vi "ECS-100X-PFI-RT.vi"() -> ()   [LabVIEW 2015]
uses:
  Typedefs/FPGA Refs/Generic FPGA Ref.ctl
  Typedefs/RT Data.ctl
  Typedefs/FPGA Refs/FPGA Refs.ctl
  Typedefs/EPT/EPT Cluster.ctl
  <vilib>/Powertrain Controls/Device Drivers/Engine Position Tracking/EPTx/RevA/RT/Controls/EPTxData.ctl
  Typedefs/Raw Inputs/Raw Inputs.ctl
  Typedefs/Raw Inputs/NI9752.ctl
  Typedefs/Raw Inputs/PPWData.ctl
  Typedefs/Raw Inputs/NI9757.ctl
  Typedefs/Raw Inputs/NI9411.ctl
  Typedefs/Raw Inputs/NI9220.ctl
  Typedefs/Raw Inputs/VRHall.ctl
  Typedefs/Control Inputs/Control Inputs.ctl
  Typedefs/EPT/Engine Status.ctl
  Typedefs/MISC/Load Control Mode.ctl
  Typedefs/Control Outputs/Control Outputs.ctl
  Typedefs/Control Outputs/Injection Quantity.ctl
  Typedefs/Control Outputs/Injection Timing.ctl
  Typedefs/Raw Outputs/Raw Outputs.ctl
  Typedefs/Raw Outputs/NI9751.ctl
  Typedefs/Raw Outputs/DI.ctl
  Typedefs/Raw Outputs/NI9754.ctl
  Typedefs/Raw Outputs/ESTTL.ctl
  Typedefs/Raw Outputs/NI9758.ctl
  Typedefs/Raw Outputs/LS.ctl
  Typedefs/Raw Outputs/PFI.ctl
  Typedefs/Raw Outputs/NI9759.ctl
  <vilib>/Platform/TimedLoop/XDataNode/timing_clust.ctl
  <vilib>/Platform/TimedLoop/XDataNode/nitl_modes.ctl
  <vilib>/Platform/TimedLoop/XDataNode/wakeup.ctl
  <vilib>/addons/Combustion Analysis System/Real-Time/Controls/Settings/CAS - Settings - Slow Speed Data.ctl
  <vilib>/addons/Combustion Analysis System/FPGA/CAS - FGPA - Reference.ctl
  Globals/DIScope Globals.vi
  <vilib>/FPGAPlugInAG/PXI-7853R/niLvFpga_Open_PXI-7853R.vi
  <vilib>/rvi/interface/common/dynamic/niFpgaDynamicAddResources.vi
  <vilib>/addons/Combustion Analysis System/Real-Time/Globals/CAS - Slow Speed Data.vi
  <vilib>/addons/Combustion Analysis System/Real-Time/Globals/Settings/CAS - Settings - Custom Properties.vi
  Globals/RT Data.vi
  <vilib>/rvi/interface/nirviOpenFPGA/nirviOpenFPGA.xnode
  FPGA Bitfiles/ECS-100X-FPGA1-EPTx.lvbitx
  FPGA Bitfiles/ECS-100X-FPGA2-EPTx.lvbitx
  <vilib>/Platform/TimedLoop/XDataNode/XDataNode.xnode
  ECS-RT.lvlib
  <vilib>/Platform/TimedLoop/XDataNode/XDNodeRunTimeDep.lvlib
  ECS-Shared.lvlib
  <vilib>/Powertrain Controls/Device Drivers/Engine Position Tracking/EPTx/RevA/RT/EPTx - RevA - RT.lvlib
panel:
  out "System Loop Iteration":i32
  in  "Stop RT":bool
  out "FPGA 2":errorcluster
  out "Slow Speed Loop Iteration":i32
  out "Iteration Duration":i64
  out "SCMInitOK":bool
  out "FPGA 1":errorcluster
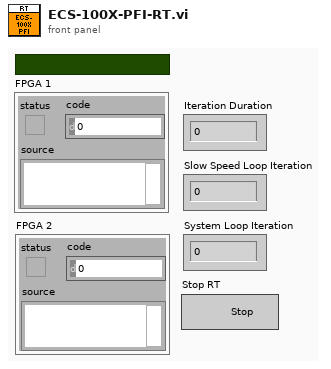
[diagram p1: front panel]
types:
  T1 = typedef "ECS-Shared.lvlib/RT Data.ctl" = cluster{"Refs":T2, "EPT":T4, "Raw Inputs":T6, "Control Inputs":T13, "Control Outputs":T16, "Raw Outputs":T19}
  T2 = typedef "ECS-Shared.lvlib/FPGA Refs.ctl" = cluster{"FPGA 1":T3, "FPGA 2":T3}
  T3 = typedef "ECS-Shared.lvlib/Generic FPGA Ref.ctl" = refnum<k20>
  T4 = typedef "ECS-Shared.lvlib/EPT Cluster.ctl" = cluster{"MaxCAD":sgl, "EPT Sim Enabled":bool, "EPTxData":T5}
  T5 = typedef "EPTx - RevA - RT.lvlib/EPTxData.ctl" = cluster{"Sync":bool, "CurrentCAD":sgl, "Speed [RPM]":sgl, "Config":bool, "Rcvg Primary":bool, "Stall":bool, "Overflow":bool, "Ratio Error":bool, "Pattern Error":bool, "Aux Warning":bool, "Watchdog Error":bool}
  T6 = typedef "ECS-Shared.lvlib/Raw Inputs.ctl" = cluster{"NI9752s":T7[], "NI9757s":T9[], "NI9411s":T10[], "NI9220s":T11[], "VRHalls":T12[]}
  T7 = typedef "ECS-Shared.lvlib/NI9752.ctl" = cluster{"Voltage [V]":sgl[], "Resistance [Ohm]":sgl[], "PPWData VR1":T8, "PPWData VR2":T8, "PPWData Hall1":T8, "PPWData Hall2":T8}
  T8 = typedef "ECS-Shared.lvlib/PPWData.ctl" = cluster{"Period":u32, "PulseWidth":u32, "Stopped":bool}
  T9 = typedef "ECS-Shared.lvlib/NI9757.ctl" = cluster{"UEGO1":cluster{"Lambda":sgl, "Phi":sgl, "AF_Ratio":sgl, "Ip":sgl, "Temp":sgl, "Hot":bool}, "UEGO2":cluster{"Lambda":sgl, "Phi":sgl, "AF_Ratio":sgl, "Ip":sgl, "Temp":sgl, "Hot":bool}, "EGO1":cluster{"Status":enum16{"COLD SENSOR", "FOULED SENSOR", "RICH", "LEAN"}, "SensorV":sgl}, "EGO2":cluster{"Status":enum16{"COLD SENSOR", "FOULED SENSOR", "RICH", "LEAN"}, "SensorV":sgl}, "EGO3":cluster{"Status":enum16{"COLD SENSOR", "FOULED SENSOR", "RICH", "LEAN"}, "SensorV":sgl}, "EGO4":cluster{"Status":enum16{"COLD SENSOR", "FOULED SENSOR", "RICH", "LEAN"}, "SensorV":sgl}}
  T10 = typedef "ECS-Shared.lvlib/NI9411.ctl" = cluster{"PPWData 0":T8, "PPWData 1":T8, "PPWData 2":T8, "PPWData 3":T8, "PPWData 4":T8, "PPWData 5":T8}
  T11 = typedef "ECS-Shared.lvlib/NI9220.ctl" = cluster{"AI 0":sgl, "AI 1":sgl, "AI 2":sgl, "AI 3":sgl, "AI 4":sgl, "AI 5":sgl, "AI 6":sgl, "AI 7":sgl, "AI 8":sgl, "AI 9":sgl, "AI 10":sgl, "AI 11":sgl, "AI 12":sgl, "AI 13":sgl, "AI 14":sgl, "AI 15":sgl}
  T12 = typedef "ECS-Shared.lvlib/VRHall.ctl" = cluster{"PPWData 0":T8, "PPWData 1":T8, "PPWData 2":T8, "PPWData 3":T8, "PPWData 4":T8, "PPWData 5":T8}
  T13 = typedef "ECS-Shared.lvlib/Control Inputs.ctl" = cluster{"Engine Speed [RPM]":sgl, "Engine Status":T14, "Load Control \nMode":T15, "dt(s)":sgl, "Number of Cylinders":u8, "Engine Displacement [cc]":sgl, "StoichAFR":sgl, "Q.LHV Fuel [kJ/kg]":sgl, "BattV PSU [V]":sgl, "12V PSU [V]":sgl, "5V PSU [V]":sgl, "Pedal Position [%]":sgl, "Oil Pressure [kPa]":sgl, "Oil Temp [C]":sgl, "Oil Level [%]":sgl, "Engine Coolant Temp (ECT) [C]":sgl, "Engine Coolant Pressure [kPa]":sgl, "Rail Pressure [bar]":sgl, "Fuel Pressure [kPa]":sgl, "Fuel Temp [C]":sgl, "Vacuum Pressure [kPa]":sgl, "Throttle Position [%]":sgl, "Cam1 Advance [CAD]":sgl, "Cam2 Advance [CAD]":sgl, "Cam3 Advance [CAD]":sgl, "Cam4 Advance [CAD]":sgl, "CA50 Control Output [CAD]":sgl[], "CA50 Control Output Valid":bool[], "Intake Air Temp (IAT) [C]":sgl, "Barometric Air Pressure [kPa]":sgl, "Intake Air Rel. Humidity [%]":sgl, "Mass Air Flow (MAF) [kg/hr]":sgl, "Turbo Inlet Air Pressure [kPa]":sgl, "Turbo Inlet Air Temp [C]":sgl, "Turbo Outlet Air Pressure [kPa]":sgl, "Turbo Outlet Air Temp [C]":sgl, "CAC Outlet Pressure [kPa]":sgl, "CAC Outlet Temp [C]":sgl, "Intake Manifold Pressure (MAP) [kPa]":sgl, "Intake Manifold Temp (MAT) [C]":sgl, "Exhaust Manifold Pressure [kPa]":sgl, "Exhaust Manifold Temp [C]":sgl, "HighP EGR Cooler Outlet Pressure [kPa]":sgl, "HighP EGR Cooler Outlet Temp [C]":sgl, "HighP EGR Differential Pressure [kPa]":sgl, "HighP EGR Valve Position [%]":sgl, "Turbo Outlet Exhaust Pressure [kPa]":sgl, "Turbo Outlet Exhaust Temp [C]":sgl, "VGT Position 1 [%]":sgl, "VGT Position 2 [%]":sgl, "Turbo Speed 1 [RPM]":sgl, "Turbo Speed 2 [RPM]":sgl, "LowP EGR Differential Pressure [kPa]":sgl, "LowP EGR Valve Position [%]":sgl, "UEGO1Lambda":sgl, "UEGO1_Hot":bool, "UEGO2Lambda":sgl, "UEGO2_Hot":bool, "Knock Intensity":sgl[], "Knock":bool[]}
  T14 = typedef "ECS-Shared.lvlib/Engine Status.ctl" = enum16{"OFF", "STALLED", "CRANKING", "RUNNING", "ACCEL", "DECEL", "SAFE"}
  T15 = typedef "ECS-Shared.lvlib/Load Control Mode.ctl" = enum16{"No Governor", "Low-Idle Governor", "High-Idle Governor"}
  T16 = typedef "ECS-Shared.lvlib/Control Outputs.ctl" = cluster{"Pedal Desired [%]":sgl, "MEP Desired [bar]":sgl, "Fuel Desired [mg/cyc]":sgl, "Intake MAP Desired [kPa]":sgl, "Cam1 Advance Setpoint [CAD]":sgl, "Cam2 Advance Setpoint [CAD]":sgl, "HighP EGR Position Setpoint [%Open]":sgl, "LowP EGR Position Setpoint [%Open]":sgl, "Rail Pressure Setpoint [bar]":sgl, "Wastegate1 Position Setpoint [%Open]":sgl, "Wastegate2 Position Setpoint [%Open]":sgl, "VGT1 Position Setpoint [%Open]":sgl, "VGT2 Position Setpoint [%Open]":sgl, "Throttle1 Position Setpoint [%Open]":sgl, "Throttle2 Position Setpoint [%Open]":sgl, "TurboBPV Position Setpoint [%Open]":sgl, "Spark Dwells [msec]":sgl[], "Spark Timings [DBTDC]":sgl[], "PFI Quantities [mg/inj]":sgl[], "PFI Timings [DBTDC]":sgl[], "DI Quantities [mg/inj]":T17[], "DI Timings [DBTDC]":T18[]}
  T17 = typedef "ECS-Shared.lvlib/Injection Quantity.ctl" = cluster{"Pilot1Quantity [mg/inj]":sgl, "Pilot2Quantity [mg/inj]":sgl, "MainQuantity [mg/inj]":sgl, "Post1Quantity [mg/inj]":sgl, "Post2Quantity [mg/inj]":sgl}
  T18 = typedef "ECS-Shared.lvlib/Injection Timing.ctl" = cluster{"Pilot1SOI [DBTDC]":sgl, "Pilot2SOI [DBTDC]":sgl, "MainSOI [DBTDC]":sgl, "Post1SOI [DBTDC]":sgl, "Post2SOI [DBTDC]":sgl}
  T19 = typedef "ECS-Shared.lvlib/Raw Outputs.ctl" = cluster{"9751-1":T20, "9751-2":T20, "9751-3":T20, "9751-4":T20, "9754-1":T22, "9754-2":T22, "9758-1":T24, "9758-2":T24, "9759-1":T27}
  T20 = typedef "ECS-Shared.lvlib/NI9751.ctl" = cluster{"DI1":T21, "DI2":T21, "DI3":T21}
  T21 = typedef "ECS-Shared.lvlib/DI.ctl" = cluster{"Window_Start (DBTDC)":sgl, "Window_End (DBTDC)":sgl, "Enable_Inj1":bool, "Duration_Inj1 (msec)":sgl, "Timing_Inj1 (DBTDC)":sgl, "Enable_Inj2":bool, "Duration_Inj2 (msec)":sgl, "Timing_Inj2 (DBTDC)":sgl, "Enable_Inj3":bool, "Duration_Inj3 (msec)":sgl, "Timing_Inj3 (DBTDC)":sgl, "Enable_Inj4":bool, "Duration_Inj4 (msec)":sgl, "Timing_Inj4 (DBTDC)":sgl, "Enable_Inj5":bool, "Duration_Inj5 (msec)":sgl, "Timing_Inj5 (DBTDC)":sgl}
  T22 = typedef "ECS-Shared.lvlib/NI9754.ctl" = cluster{"ESTTL 1":T23, "ESTTL 2":T23, "ESTTL 3":T23, "ESTTL 4":T23, "ESTTL 5":T23, "ESTTL 6":T23, "ESTTL 7":T23, "ESTTL 8":T23}
  T23 = typedef "ECS-Shared.lvlib/ESTTL.ctl" = cluster{"Timing (DBTDC)":sgl, "Dwell (ms)":sgl}
  T24 = typedef "ECS-Shared.lvlib/NI9758.ctl" = cluster{"LS 1":T25, "LS 2":T25, "LS 3":T25, "LS 4":T25, "PFI 1":T26, "PFI 2":T26, "PFI 3":T26, "PFI 4":T26}
  T25 = typedef "ECS-Shared.lvlib/LS.ctl" = cluster{"Enable":bool, "Freq [Hz]":sgl, "DutyCyc [%]":sgl}
  T26 = typedef "ECS-Shared.lvlib/PFI.ctl" = cluster{"Position Mode":bool, "Timing (DBTDC)":sgl, "Pulse Width (ms)":sgl}
  T27 = typedef "ECS-Shared.lvlib/NI9759.ctl" = cluster{"THR1-1 DC [%]":sgl, "THR1-1 Setpoint [% Open]":sgl, "THR1-2 DC [%]":sgl, "THR1-2 Setpoint [% Open]":sgl}
  T28 = typedef "CAS - FGPA - Reference.ctl" = refnum<k20>
  T29 = typedef "XDNodeRunTimeDep.lvlib/timing_clust.ctl" = cluster{"Expected End [f-1]":u64, "Actual End [f-1]":u64, "Finished Late? [f-1]":bool, "Expected End [i-1]":u64, "Actual End [i-1]":u64, "Finished Late? [i-1]":bool, "Expected Start [i]":u64, "Actual Start [i]":u64, "Expected Start [f]":u64, "Actual Start [f]":u64, "Source Name":string, "Structure Name":string, "Period":i64, "Deadline":i64, "Offset":i64, "Start":i64, "Priority":i32, "Timeout":i32, "Mode":T30, "Wakeup Reason":T31, "Error":errorcluster, "Source Type":string, "Secondary Source Type":string, "Global End Time":u64, "Global Start Time":u64, "Frame Duration":u64, "Iteration Duration":u64, "Assigned CPU":i32, "I/O Scan Engine Mode":u32}
  T30 = typedef "XDNodeRunTimeDep.lvlib/nitl_modes.ctl" = enum32{"No Change", "Process missed periods, maintain original phase", "Discard missed periods, maintain original phase", "Process missed periods, ignore original phase", "Discard missed periods, ignore original phase"}
  T31 = typedef "XDNodeRunTimeDep.lvlib/wakeup.ctl" = enum32{"Normal", "Aborted", "Asynchronous wakeup", "Timing source error", "Timed loop error", "Timeout"}
  T32 = typedef "CAS - Settings - Slow Speed Data.ctl" = cluster{"Name":string, "Units":string, "Value":sgl}
  T33 = typedef "CAS - Settings - Custom Properities.ctl" = T34[]
  T34 = typedef "CAS - Settings - Custom Properity.ctl" = cluster{"Properity":string, "Data":string}
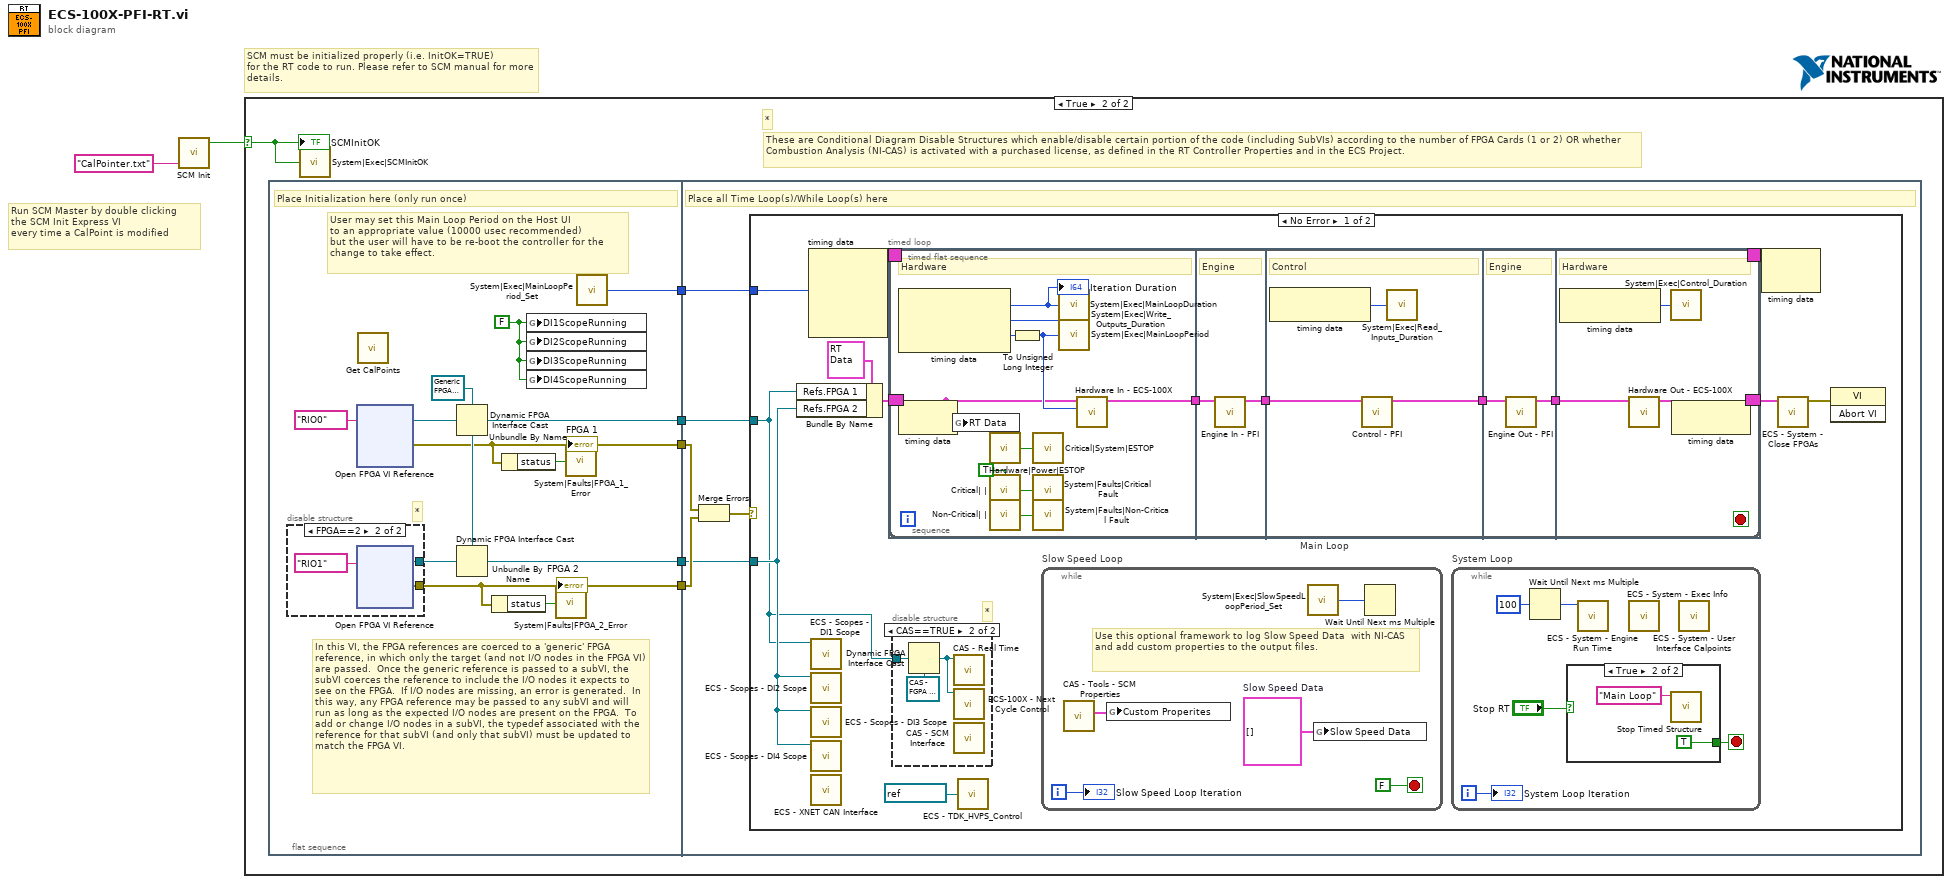
[diagram p0: block diagram]
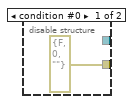
[diagram p3: hidden frame]
diagram:
  # "SCM must be initialized properly (i.e. InitOK=TRUE)\nfor the RT code to run. Please refer to SCM manual for more details."
  # "Run SCM Master by double clicking\nthe SCM Init Express VI\nevery time a CalPoint is modified"
  n1 = call "SCM Init"("Calibration File"="CalPointer.txt") -> ("InitOK"=w2:bool)  [unwired: 2 in, 2 out]
  n2 = case shown="True" w2 {
    selector: w2 -> [_ w8]
    frame False {
    }
    frame True {
      # "These are Conditional Diagram Disable Structures which enable/disable certain portion of the code (including SubVIs) according to the number of FPGA Cards (1 or 2) OR whether Combustion Analysis (NI-CAS) is activated with a purchased license, as defined in the RT Controller Properties and in the ECS Project."
      # "*"
      n3 = flat-sequence {
        tunnel: [w9] -> w7
        tunnel: [w16] -> w6
        tunnel: [w19] -> w5
        tunnel: [w15] -> w4
        tunnel: [w12] -> w3
        tunnel: w7 -> [w30]
        tunnel: w6 -> [w29]
        tunnel: w5 -> [w27]
        tunnel: w4 -> [w26]
        tunnel: w3 -> [w25]
        frame #0 {
          w13 = T3 refnum ("FPGA VI Reference Out")
          w18 = FALSE ("DIScopeTransfer")
          # "*"
          # "In this VI, the FPGA references are coerced to a 'generic' FPGA reference, in which only the target (and not I/O nodes in the FPGA VI) are passed.  Once the generic reference is passed to a subVI, the subVI coerces the reference to include the I/O nodes it expects to see on the FPGA.  If I/O nodes are missing, an error is generated.  In this way, any FPGA reference may be passed to any subVI and will run as long as the expected I/O nodes are present on the FPGA.  To add or change I/O nodes in a subVI, the typedef associated with the reference for that subVI (and only that subVI) must be updated to match the FPGA VI."
          # "User may set this Main Loop Period on the Host UI\nto an appropriate value (10000 usec recommended)\nbut the user will have to be re-boot the controller for the\nchange to take effect."
          # "Place Initialization here (only run once)"
          n4 = disable-structure shown="FPGA==2" {
            disable-tunnel: [errorcluster {"status"=FALSE, "code"=0, "source"=""} ("error out") w23] -> w16
            disable-tunnel: [_ w22] -> w14
            frame condition #0 {
            }
            frame condition #1 (active) {
              n5 = xnode "Open FPGA VI Reference"("resource name"=tag "RIO1") -> ("FPGA VI Reference Out"=w22:refnum<k20>, "error out"=w23:errorcluster)  [unwired: 1 in]
            }
          }
          "FPGA 2" <- w16
          n6 = xnode "Open FPGA VI Reference"("resource name"=tag "RIO0") -> ("FPGA VI Reference Out"=w10:refnum<k20>, "error out"=w9:errorcluster)  [unwired: 1 in]
          "FPGA 1" <- w9
          n7 = call "Get CalPoints.vi"() -> ()  [unwired: 12 in]
          n8 = Dynamic FPGA Interface Cast(Session In=w13, Type=w10) -> (Session Out=w15:T3)
          n9 = Dynamic FPGA Interface Cast(Session In=w13, Type=w14) -> (Session Out=w12:T3)
          n10 = Unbundle By Name(w16) -> ("status"=w17:bool)
          n11 = Unbundle By Name(w9) -> ("status"=w20:bool)
          n12 = global write "DIScope Globals.vi" "DI1ScopeRunning"(w18) -> ()
          n13 = global write "DIScope Globals.vi" "DI2ScopeRunning"(w18) -> ()
          n14 = global write "DIScope Globals.vi" "DI3ScopeRunning"(w18) -> ()
          n15 = global write "DIScope Globals.vi" "DI4ScopeRunning"(w18) -> ()
          n16 = call "System|Faults|FPGA_2_Error"("Value"=w17) -> ()
          n17 = call "System|Faults|FPGA_1_Error"("Value"=w20) -> ()
          n18 = call "System|Exec|MainLoopPeriod_Set"() -> ("Value"=w19:u32)
        }
        frame #1 {
          # "Place all Time Loop(s)/While Loop(s) here"
          n19 = Merge Errors(w30, w29) -> (w28:errorcluster)
          n20 = case shown="No Error" w28 {
            tunnel: w27 -> [w38 _]
            tunnel: w26 -> [w33 _]
            tunnel: w25 -> [w35 _]
            frame No Error {
              # "*"
              n21 = Bundle By Name(cluster=T1 {"Refs"={"FPGA 1"=refnum, "FPGA 2"=refnum}, "EPT"={"MaxCAD"=0.0, "EPT Sim Enabled"=FALSE, "EPTxData"={"Sync"=FALSE, "CurrentCAD"=0.0, "Speed [RPM]"=0.0, "Config"=FALSE, "Rcvg Primary"=FALSE, "Stall"=FALSE, "Overflow"=FALSE, "Ratio Error"=FALSE, "Pattern Error"=FALSE, "Aux Warning"=FALSE, "Watchdog Error"=FALSE}}, "Raw Inputs"={"NI9752s"=[], "NI9757s"=[], "NI9411s"=[], "NI9220s"=[], "VRHalls"=[]}, "Control Inputs"={"Engine Speed [RPM]"=0.0, "Engine Status"=enum."STALLED", "Load Control \nMode"=enum."No Governor", "dt(s)"=0.0, "Number of Cylinders"=0, "Engine Displacement [cc]"=0.0, "StoichAFR"=0.0, "Q.LHV Fuel [kJ/kg]"=0.0, "BattV PSU [V]"=0.0, "12V PSU [V]"=0.0, "5V PSU [V]"=0.0, "Pedal Position [%]"=0.0, "Oil Pressure [kPa]"=0.0, "Oil Temp [C]"=0.0, "Oil Level [%]"=0.0, "Engine Coolant Temp (ECT) [C]"=0.0, "Engine Coolant Pressure [kPa]"=0.0, "Rail Pressure [bar]"=0.0, "Fuel Pressure [kPa]"=0.0, "Fuel Temp [C]"=0.0, "Vacuum Pressure [kPa]"=0.0, "Throttle Position [%]"=0.0, "Cam1 Advance [CAD]"=0.0, "Cam2 Advance [CAD]"=0.0, "Cam3 Advance [CAD]"=0.0, "Cam4 Advance [CAD]"=0.0, "CA50 Control Output [CAD]"=[], "CA50 Control Output Valid"=[], "Intake Air Temp (IAT) [C]"=0.0, "Barometric Air Pressure [kPa]"=0.0, "Intake Air Rel. Humidity [%]"=0.0, "Mass Air Flow (MAF) [kg/hr]"=0.0, "Turbo Inlet Air Pressure [kPa]"=0.0, "Turbo Inlet Air Temp [C]"=0.0, "Turbo Outlet Air Pressure [kPa]"=0.0, "Turbo Outlet Air Temp [C]"=0.0, "CAC Outlet Pressure [kPa]"=0.0, "CAC Outlet Temp [C]"=0.0, "Intake Manifold Pressure (MAP) [kPa]"=0.0, "Intake Manifold Temp (MAT) [C]"=0.0, "Exhaust Manifold Pressure [kPa]"=0.0, "Exhaust Manifold Temp [C]"=0.0, "HighP EGR Cooler Outlet Pressure [kPa]"=0.0, "HighP EGR Cooler Outlet Temp [C]"=0.0, "HighP EGR Differential Pressure [kPa]"=0.0, "HighP EGR Valve Position [%]"=0.0, "Turbo Outlet Exhaust Pressure [kPa]"=0.0, "Turbo Outlet Exhaust Temp [C]"=0.0, "VGT Position 1 [%]"=0.0, "VGT Position 2 [%]"=0.0, "Turbo Speed 1 [RPM]"=0.0, "Turbo Speed 2 [RPM]"=0.0, "LowP EGR Differential Pressure [kPa]"=0.0, "LowP EGR Valve Position [%]"=0.0, "UEGO1Lambda"=0.0, "UEGO1_Hot"=FALSE, "UEGO2Lambda"=0.0, "UEGO2_Hot"=FALSE, "Knock Intensity"=[], "Knock"=[]}, "Control Outputs"={"Pedal Desired [%]"=0.0, "MEP Desired [bar]"=0.0, "Fuel Desired [mg/cyc]"=0.0, "Intake MAP Desired [kPa]"=0.0, "Cam1 Advance Setpoint [CAD]"=0.0, "Cam2 Advance Setpoint [CAD]"=0.0, "HighP EGR Position Setpoint [%Open]"=0.0, "LowP EGR Position Setpoint [%Open]"=0.0, "Rail Pressure Setpoint [bar]"=0.0, "Wastegate1 Position Setpoint [%Open]"=0.0, "Wastegate2 Position Setpoint [%Open]"=0.0, "VGT1 Position Setpoint [%Open]"=0.0, "VGT2 Position Setpoint [%Open]"=0.0, "Throttle1 Position Setpoint [%Open]"=0.0, "Throttle2 Position Setpoint [%Open]"=0.0, "TurboBPV Position Setpoint [%Open]"=0.0, "Spark Dwells [msec]"=[], "Spark Timings [DBTDC]"=[], "PFI Quantities [mg/inj]"=[], "PFI Timings [DBTDC]"=[], "DI Quantities [mg/inj]"=[], "DI Timings [DBTDC]"=[]}, "Raw Outputs"={"9751-1"={"DI1"={"Window_Start (DBTDC)"=0.0, "Window_End (DBTDC)"=0.0, "Enable_Inj1"=FALSE, "Duration_Inj1 (msec)"=0.0, "Timing_Inj1 (DBTDC)"=0.0, "Enable_Inj2"=FALSE, "Duration_Inj2 (msec)"=0.0, "Timing_Inj2 (DBTDC)"=0.0, "Enable_Inj3"=FALSE, "Duration_Inj3 (msec)"=0.0, "Timing_Inj3 (DBTDC)"=0.0, "Enable_Inj4"=FALSE, "Duration_Inj4 (msec)"=0.0, "Timing_Inj4 (DBTDC)"=0.0, "Enable_Inj5"=FALSE, "Duration_Inj5 (msec)"=0.0, "Timing_Inj5 (DBTDC)"=0.0}, "DI2"={"Window_Start (DBTDC)"=0.0, "Window_End (DBTDC)"=0.0, "Enable_Inj1"=FALSE, "Duration_Inj1 (msec)"=0.0, "Timing_Inj1 (DBTDC)"=0.0, "Enable_Inj2"=FALSE, "Duration_Inj2 (msec)"=0.0, "Timing_Inj2 (DBTDC)"=0.0, "Enable_Inj3"=FALSE, "Duration_Inj3 (msec)"=0.0, "Timing_Inj3 (DBTDC)"=0.0, "Enable_Inj4"=FALSE, "Duration_Inj4 (msec)"=0.0, "Timing_Inj4 (DBTDC)"=0.0, "Enable_Inj5"=FALSE, "Duration_Inj5 (msec)"=0.0, "Timing_Inj5 (DBTDC)"=0.0}, "DI3"={"Window_Start (DBTDC)"=0.0, "Window_End (DBTDC)"=0.0, "Enable_Inj1"=FALSE, "Duration_Inj1 (msec)"=0.0, "Timing_Inj1 (DBTDC)"=0.0, "Enable_Inj2"=FALSE, "Duration_Inj2 (msec)"=0.0, "Timing_Inj2 (DBTDC)"=0.0, "Enable_Inj3"=FALSE, "Duration_Inj3 (msec)"=0.0, "Timing_Inj3 (DBTDC)"=0.0, "Enable_Inj4"=FALSE, "Duration_Inj4 (msec)"=0.0, "Timing_Inj4 (DBTDC)"=0.0, "Enable_Inj5"=FALSE, "Duration_Inj5 (msec)"=0.0, "Timing_Inj5 (DBTDC)"=0.0}}, "9751-2"={"DI1"={"Window_Start (DBTDC)"=0.0, "Window_End (DBTDC)"=0.0, "Enable_Inj1"=FALSE, "Duration_Inj1 (msec)"=0.0, "Timing_Inj1 (DBTDC)"=0.0, "Enable_Inj2"=FALSE, "Duration_Inj2 (msec)"=0.0, "Timing_Inj2 (DBTDC)"=0.0, "Enable_Inj3"=FALSE, "Duration_Inj3 (msec)"=0.0, "Timing_Inj3 (DBTDC)"=0.0, "Enable_Inj4"=FALSE, "Duration_Inj4 (msec)"=0.0, "Timing_Inj4 (DBTDC)"=0.0, "Enable_Inj5"=FALSE, "Duration_Inj5 (msec)"=0.0, "Timing_Inj5 (DBTDC)"=0.0}, "DI2"={"Window_Start (DBTDC)"=0.0, "Window_End (DBTDC)"=0.0, "Enable_Inj1"=FALSE, "Duration_Inj1 (msec)"=0.0, "Timing_Inj1 (DBTDC)"=0.0, "Enable_Inj2"=FALSE, "Duration_Inj2 (msec)"=0.0, "Timing_Inj2 (DBTDC)"=0.0, "Enable_Inj3"=FALSE, "Duration_Inj3 (msec)"=0.0, "Timing_Inj3 (DBTDC)"=0.0, "Enable_Inj4"=FALSE, "Duration_Inj4 (msec)"=0.0, "Timing_Inj4 (DBTDC)"=0.0, "Enable_Inj5"=FALSE, "Duration_Inj5 (msec)"=0.0, "Timing_Inj5 (DBTDC)"=0.0}, "DI3"={"Window_Start (DBTDC)"=0.0, "Window_End (DBTDC)"=0.0, "Enable_Inj1"=FALSE, "Duration_Inj1 (msec)"=0.0, "Timing_Inj1 (DBTDC)"=0.0, "Enable_Inj2"=FALSE, "Duration_Inj2 (msec)"=0.0, "Timing_Inj2 (DBTDC)"=0.0, "Enable_Inj3"=FALSE, "Duration_Inj3 (msec)"=0.0, "Timing_Inj3 (DBTDC)"=0.0, "Enable_Inj4"=FALSE, "Duration_Inj4 (msec)"=0.0, "Timing_Inj4 (DBTDC)"=0.0, "Enable_Inj5"=FALSE, "Duration_Inj5 (msec)"=0.0, "Timing_Inj5 (DBTDC)"=0.0}}, "9751-3"={"DI1"={"Window_Start (DBTDC)"=0.0, "Window_End (DBTDC)"=0.0, "Enable_Inj1"=FALSE, "Duration_Inj1 (msec)"=0.0, "Timing_Inj1 (DBTDC)"=0.0, "Enable_Inj2"=FALSE, "Duration_Inj2 (msec)"=0.0, "Timing_Inj2 (DBTDC)"=0.0, "Enable_Inj3"=FALSE, "Duration_Inj3 (msec)"=0.0, "Timing_Inj3 (DBTDC)"=0.0, "Enable_Inj4"=FALSE, "Duration_Inj4 (msec)"=0.0, "Timing_Inj4 (DBTDC)"=0.0, "Enable_Inj5"=FALSE, "Duration_Inj5 (msec)"=0.0, "Timing_Inj5 (DBTDC)"=0.0}, "DI2"={"Window_Start (DBTDC)"=0.0, "Window_End (DBTDC)"=0.0, "Enable_Inj1"=FALSE, "Duration_Inj1 (msec)"=0.0, "Timing_Inj1 (DBTDC)"=0.0, "Enable_Inj2"=FALSE, "Duration_Inj2 (msec)"=0.0, "Timing_Inj2 (DBTDC)"=0.0, "Enable_Inj3"=FALSE, "Duration_Inj3 (msec)"=0.0, "Timing_Inj3 (DBTDC)"=0.0, "Enable_Inj4"=FALSE, "Duration_Inj4 (msec)"=0.0, "Timing_Inj4 (DBTDC)"=0.0, "Enable_Inj5"=FALSE, "Duration_Inj5 (msec)"=0.0, "Timing_Inj5 (DBTDC)"=0.0}, "DI3"={"Window_Start (DBTDC)"=0.0, "Window_End (DBTDC)"=0.0, "Enable_Inj1"=FALSE, "Duration_Inj1 (msec)"=0.0, "Timing_Inj1 (DBTDC)"=0.0, "Enable_Inj2"=FALSE, "Duration_Inj2 (msec)"=0.0, "Timing_Inj2 (DBTDC)"=0.0, "Enable_Inj3"=FALSE, "Duration_Inj3 (msec)"=0.0, "Timing_Inj3 (DBTDC)"=0.0, "Enable_Inj4"=FALSE, "Duration_Inj4 (msec)"=0.0, "Timing_Inj4 (DBTDC)"=0.0, "Enable_Inj5"=FALSE, "Duration_Inj5 (msec)"=0.0, "Timing_Inj5 (DBTDC)"=0.0}}, "9751-4"={"DI1"={"Window_Start (DBTDC)"=0.0, "Window_End (DBTDC)"=0.0, "Enable_Inj1"=FALSE, "Duration_Inj1 (msec)"=0.0, "Timing_Inj1 (DBTDC)"=0.0, "Enable_Inj2"=FALSE, "Duration_Inj2 (msec)"=0.0, "Timing_Inj2 (DBTDC)"=0.0, "Enable_Inj3"=FALSE, "Duration_Inj3 (msec)"=0.0, "Timing_Inj3 (DBTDC)"=0.0, "Enable_Inj4"=FALSE, "Duration_Inj4 (msec)"=0.0, "Timing_Inj4 (DBTDC)"=0.0, "Enable_Inj5"=FALSE, "Duration_Inj5 (msec)"=0.0, "Timing_Inj5 (DBTDC)"=0.0}, "DI2"={"Window_Start (DBTDC)"=0.0, "Window_End (DBTDC)"=0.0, "Enable_Inj1"=FALSE, "Duration_Inj1 (msec)"=0.0, "Timing_Inj1 (DBTDC)"=0.0, "Enable_Inj2"=FALSE, "Duration_Inj2 (msec)"=0.0, "Timing_Inj2 (DBTDC)"=0.0, "Enable_Inj3"=FALSE, "Duration_Inj3 (msec)"=0.0, "Timing_Inj3 (DBTDC)"=0.0, "Enable_Inj4"=FALSE, "Duration_Inj4 (msec)"=0.0, "Timing_Inj4 (DBTDC)"=0.0, "Enable_Inj5"=FALSE, "Duration_Inj5 (msec)"=0.0, "Timing_Inj5 (DBTDC)"=0.0}, "DI3"={"Window_Start (DBTDC)"=0.0, "Window_End (DBTDC)"=0.0, "Enable_Inj1"=FALSE, "Duration_Inj1 (msec)"=0.0, "Timing_Inj1 (DBTDC)"=0.0, "Enable_Inj2"=FALSE, "Duration_Inj2 (msec)"=0.0, "Timing_Inj2 (DBTDC)"=0.0, "Enable_Inj3"=FALSE, "Duration_Inj3 (msec)"=0.0, "Timing_Inj3 (DBTDC)"=0.0, "Enable_Inj4"=FALSE, "Duration_Inj4 (msec)"=0.0, "Timing_Inj4 (DBTDC)"=0.0, "Enable_Inj5"=FALSE, "Duration_Inj5 (msec)"=0.0, "Timing_Inj5 (DBTDC)"=0.0}}, "9754-1"={"ESTTL 1"={"Timing (DBTDC)"=0.0, "Dwell (ms)"=0.0}, "ESTTL 2"={"Timing (DBTDC)"=0.0, "Dwell (ms)"=0.0}, "ESTTL 3"={"Timing (DBTDC)"=0.0, "Dwell (ms)"=0.0}, "ESTTL 4"={"Timing (DBTDC)"=0.0, "Dwell (ms)"=0.0}, "ESTTL 5"={"Timing (DBTDC)"=0.0, "Dwell (ms)"=0.0}, "ESTTL 6"={"Timing (DBTDC)"=0.0, "Dwell (ms)"=0.0}, "ESTTL 7"={"Timing (DBTDC)"=0.0, "Dwell (ms)"=0.0}, "ESTTL 8"={"Timing (DBTDC)"=0.0, "Dwell (ms)"=0.0}}, "9754-2"={"ESTTL 1"={"Timing (DBTDC)"=0.0, "Dwell (ms)"=0.0}, "ESTTL 2"={"Timing (DBTDC)"=0.0, "Dwell (ms)"=0.0}, "ESTTL 3"={"Timing (DBTDC)"=0.0, "Dwell (ms)"=0.0}, "ESTTL 4"={"Timing (DBTDC)"=0.0, "Dwell (ms)"=0.0}, "ESTTL 5"={"Timing (DBTDC)"=0.0, "Dwell (ms)"=0.0}, "ESTTL 6"={"Timing (DBTDC)"=0.0, "Dwell (ms)"=0.0}, "ESTTL 7"={"Timing (DBTDC)"=0.0, "Dwell (ms)"=0.0}, "ESTTL 8"={"Timing (DBTDC)"=0.0, "Dwell (ms)"=0.0}}, "9758-1"={"LS 1"={"Enable"=FALSE, "Freq [Hz]"=0.0, "DutyCyc [%]"=0.0}, "LS 2"={"Enable"=FALSE, "Freq [Hz]"=0.0, "DutyCyc [%]"=0.0}, "LS 3"={"Enable"=FALSE, "Freq [Hz]"=0.0, "DutyCyc [%]"=0.0}, "LS 4"={"Enable"=FALSE, "Freq [Hz]"=0.0, "DutyCyc [%]"=0.0}, "PFI 1"={"Position Mode"=FALSE, "Timing (DBTDC)"=0.0, "Pulse Width (ms)"=0.0}, "PFI 2"={"Position Mode"=FALSE, "Timing (DBTDC)"=0.0, "Pulse Width (ms)"=0.0}, "PFI 3"={"Position Mode"=FALSE, "Timing (DBTDC)"=0.0, "Pulse Width (ms)"=0.0}, "PFI 4"={"Position Mode"=FALSE, "Timing (DBTDC)"=0.0, "Pulse Width (ms)"=0.0}}, "9758-2"={"LS 1"={"Enable"=FALSE, "Freq [Hz]"=0.0, "DutyCyc [%]"=0.0}, "LS 2"={"Enable"=FALSE, "Freq [Hz]"=0.0, "DutyCyc [%]"=0.0}, "LS 3"={"Enable"=FALSE, "Freq [Hz]"=0.0, "DutyCyc [%]"=0.0}, "LS 4"={"Enable"=FALSE, "Freq [Hz]"=0.0, "DutyCyc [%]"=0.0}, "PFI 1"={"Position Mode"=FALSE, "Timing (DBTDC)"=0.0, "Pulse Width (ms)"=0.0}, "PFI 2"={"Position Mode"=FALSE, "Timing (DBTDC)"=0.0, "Pulse Width (ms)"=0.0}, "PFI 3"={"Position Mode"=FALSE, "Timing (DBTDC)"=0.0, "Pulse Width (ms)"=0.0}, "PFI 4"={"Position Mode"=FALSE, "Timing (DBTDC)"=0.0, "Pulse Width (ms)"=0.0}}, "9759-1"={"THR1-1 DC [%]"=0.0, "THR1-1 Setpoint [% Open]"=0.0, "THR1-2 DC [%]"=0.0, "THR1-2 Setpoint [% Open]"=0.0}}} ("RT Data"), "Refs.FPGA 1"=w33, "Refs.FPGA 2"=w35) -> (w36:T1)
              n22 = node-c288(w38) -> (w40:T29)  [unwired: 3 in]
              n23 = call "ECS - Scopes - DI1 Scope.vi"("FPGA Ref"=w33) -> ()  [unwired: 11 in]
              n24 = call "ECS - Scopes - DI2 Scope.vi"("FPGA Ref"=w35) -> ()  [unwired: 11 in]
              n25 = call "ECS - Scopes - DI3 Scope.vi"("FPGA Ref"=w35) -> ()  [unwired: 11 in]
              n26 = call "ECS - Scopes - DI4 Scope.vi"("FPGA Ref"=w35) -> ()  [unwired: 11 in]
              n27 = call "ECS - XNET CAN Interface.vi"() -> ()  [unwired: 6 in]
              n28 = timed-loop "Main Loop" {
                timing: w40 -> [_]
                timing-out: [_] -> w39
                shift-right: [w57] -> w32
                shift-left: w36 -> [w56]
                stop <- _ stop-if-true
                n29 = timed-sequence {
                  timing: _ -> [_]
                  timing-out: _ -> [_]
                  tunnel: [w59] -> w57
                  tunnel: w56 -> [w58]
                  n30 = timed-flat-sequence {
                    tunnel: [w70] -> w60
                    tunnel: w58 -> [w65]
                    tunnel: [w80] -> w61
                    tunnel: w60 -> [w79]
                    tunnel: w61 -> [w83]
                    tunnel: [w84] -> w63
                    tunnel: w63 -> [w90]
                    tunnel: [w89] -> w62
                    tunnel: w62 -> [w94]
                    tunnel: [w93] -> w59
                    frame #0 {
                      w64 = TRUE ("UnAcknowledged (F)")
                      # "Hardware"
                      n31 = node-c288() -> (w73:i64, w71:i64, w72:i64)  [unwired: 1 in]
                      "Iteration Duration" <- w73
                      n32 = global write "RT Data.vi" "RT Data"(w65) -> ()
                      n33 = call "Hardware|Power|ESTOP"() -> ("Value"=w67:bool)
                      n34 = call "Critical| |"("UnAcknowledged (F)"=w64) -> ("Fault"=w68:bool)  [unwired: 1 in]
                      n35 = call "Non-Critical| |"("UnAcknowledged (F)"=w64) -> ("Fault"=w69:bool)  [unwired: 1 in]
                      n36 = To Unsigned Long Integer(number=w72) -> (unsigned 32bit integer=w66:u32)
                      n37 = call "Critical|System|ESTOP"("Fault"=w67) -> ()  [unwired: 2 in]
                      n38 = call "System|Faults|Critical Fault"("Value"=w68) -> ()
                      n39 = call "System|Faults|Non-Critical Fault"("Value"=w69) -> ()
                      n40 = call "System|Exec|MainLoopDuration"("Value"=w73) -> ()
                      n41 = call "System|Exec|Write_Outputs_Duration"("Value"=w71) -> ()
                      n42 = call "System|Exec|MainLoopPeriod"("Value"=w66) -> ()
                      n43 = call "Hardware In - ECS-100X.vi"("LoopPeriod [usec]"=w66, "RT Data in"=w65) -> ("RT Data out"=w70:T1)  [unwired: 9 in]
                    }
                    frame #1 {
                      # "Engine"
                      n44 = call "Engine In - PFI.vi"("RT Data in"=w79) -> ("RT Data out"=w80:T1)  [unwired: 10 in]
                    }
                    frame #2 {
                      # "Control"
                      n45 = node-c288() -> (w85:i64)  [unwired: 1 in]
                      n46 = call "Control - PFI.vi"("RT Data in"=w83) -> ("RT Data out"=w84:T1)  [unwired: 10 in]
                      n47 = call "System|Exec|Read_Inputs_Duration"("Value"=w85) -> ()
                    }
                    frame #3 {
                      # "Engine"
                      n48 = call "Engine Out - PFI.vi"("RT Data in"=w90) -> ("RT Data out"=w89:T1)  [unwired: 10 in]
                    }
                    frame #4 {
                      # "Hardware"
                      n49 = node-c288() -> (w95:i64)  [unwired: 1 in]
                      n50 = call "Hardware Out - ECS-100X.vi"("RT Data in"=w94) -> ("RT Data out"=w93:T1)  [unwired: 10 in]
                      n51 = call "System|Exec|Control_Duration"("Value"=w95) -> ()
                    }
                  }
                }
                n52 = node-c288() -> ()  [unwired: 1 in, 1 out]
                n53 = node-c288() -> ()  [unwired: 1 in, 1 out]
              }
              n54 = disable-structure shown="CAS==TRUE" {
                disable-tunnel: w33 -> [_ w50]
                frame condition #0 {
                }
                frame condition #1 (active) {
                  n55 = Dynamic FPGA Interface Cast(Session In=T28 refnum ("FPGA Refnum"), Type=w50) -> (Session Out=w48:T28)
                  n56 = call <vilib>:"CAS - Real Time.vi"("FPGA Refnum"=w48) -> ()  [unwired: 11 in]
                  n57 = call "ECS-100X - Next Cycle Control.vi"("CAS FPGA Ref"=w48) -> ()  [unwired: 10 in]
                  n58 = call <vilib>:"CAS - SCM Interface.vi"() -> ()  [unwired: 12 in]
                }
              }
              n59 = call "ECS - TDK_HVPS_Control.vi"("VISA In"=refnum<visa-resource-name> "COM1") -> ()  [unwired: 5 in]
              n60 = while "Slow Speed Loop" {
                i -> [w54]
                stop <- FALSE stop-if-true
                w55 = T32[] []  # Slow Speed Data
                # "Use this optional framework to log Slow Speed Data  with NI-CAS and add custom properties to the output files."
                n61 = call <vilib>:"CAS - Tools - SCM Properties.vi"() -> ("Custom Properites"=w52:T33)  [unwired: 11 in]
                n62 = global write "CAS - Settings - Custom Properties.vi" "Custom Properites"(w52) -> ()
                n63 = call "System|Exec|SlowSpeedLoopPeriod_Set"() -> ("Value"=w53:u32)
                n64 = global write "CAS - Slow Speed Data.vi" "Slow Speed Data"(w55) -> ()
                n65 = Wait Until Next ms Multiple(millisecond multiple=w53) -> ()  [unwired: 1 out]
                "Slow Speed Loop Iteration" <- w54
              }
              n66 = while "System Loop" {
                i -> [w41]
                stop <- w42 stop-if-true
                n67 = Wait Until Next ms Multiple(millisecond multiple=u32 100) -> (millisecond timer value=w45:u32)
                n68 = case shown="True" "Stop RT" {
                  tunnel: [_ TRUE] -> w42
                  frame False {
                  }
                  frame True {
                    n69 = call <vilib>:"Stop Timed Structure.vi"("name"="Main Loop") -> ()  [unwired: 10 in, 1 out]
                  }
                }
                n70 = call "ECS - System - Engine Run Time.vi"("Loop Period [ms]"=w45) -> ()  [unwired: 11 in]
                n71 = call "ECS - System - Exec Info.vi"() -> ()  [unwired: 12 in]
                n72 = call "ECS - System - User Interface Calpoints.vi"() -> ()  [unwired: 12 in]
                "System Loop Iteration" <- w41
              }
              n73 = node-c288(w39) -> ()  [unwired: 1 out]
              n74 = call "ECS - System - Close FPGAs.vi"("RT Data in"=w32) -> ("error out"=w31:errorcluster)  [unwired: 10 in]
              n75 = invoke class="VI" method="Abort VI"(error in=w31) -> ()  [unwired: 2 in, 3 out]
            }
            frame Error {
            }
          }
        }
      }
      n76 = call "System|Exec|SCMInitOK"("Value"=w8) -> ()
      "SCMInitOK" <- w8
    }
  }
